vi "Calc Type.vi"(11 "Max Calc in":refnum<class "Max Calc.lvclass">) -> (2 "Calc Type":string)   [LabVIEW 2020, in "VolatusCalcs.lvlib" / "Max Calc.lvclass"]
uses:
  Max Calc.lvclass
  Max Calc.lvclass/Max Calc.ctl
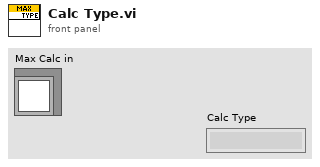
[diagram p1: front panel]
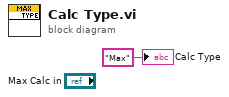
[diagram p0: block diagram]
diagram:
  "Calc Type" <- "Max" ("Calc Type")
